vi "TL midbrain THINK.vi"(0 "Forebrain Comd":T2, 3 "error in":errorcluster, 4 "IR Sensors":T1) -> (5 "Behavior arrays":T3, 6 "Behavior\nVelocity OUT":dbl, 7 "error out":errorcluster)   [LabVIEW 2014]
doc: "This vi is the midbrain THINK routine. It selects the behaviors which the boat will use based upon the passed Forebrain Command."
uses:
  sensorsSTD.ctl
panel:
  out "Waveform Graph":cluster{dbl, dbl, dbl[][]}(graph)
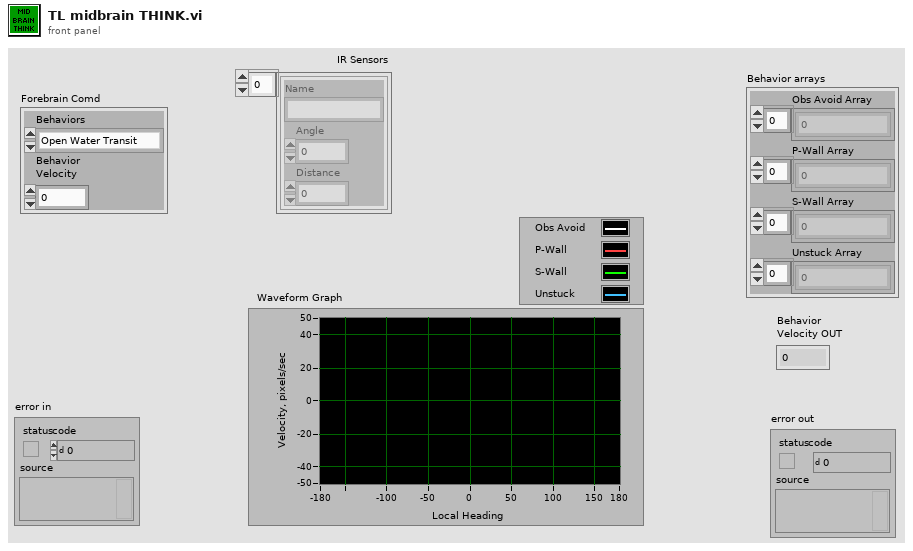
[diagram p1: front panel]
types:
  T1 = typedef "sensorsSTD.ctl" = cluster{"Name":string, "Angle":dbl, "Distance":dbl}[]
  T2 = cluster{"Behaviors":enum16{"Open Water Transit", "P-Wall Follow", "S-Wall Follow", "Get Unstuck"}, "Behavior\nVelocity":dbl}
  T3 = cluster{"Obs Avoid Array":dbl[], "P-Wall Array":dbl[], "S-Wall Array":dbl[], "Unstuck Array":dbl[]}
  T4 = enum16{"Open Water Transit", "P-Wall Follow", "S-Wall Follow", "Get Unstuck"}
  T5 = cluster{"Obstacle Avoidance":bool, "P-Wall Follow":bool, "S-Wall Follow":bool, "Get Unstuck":bool}
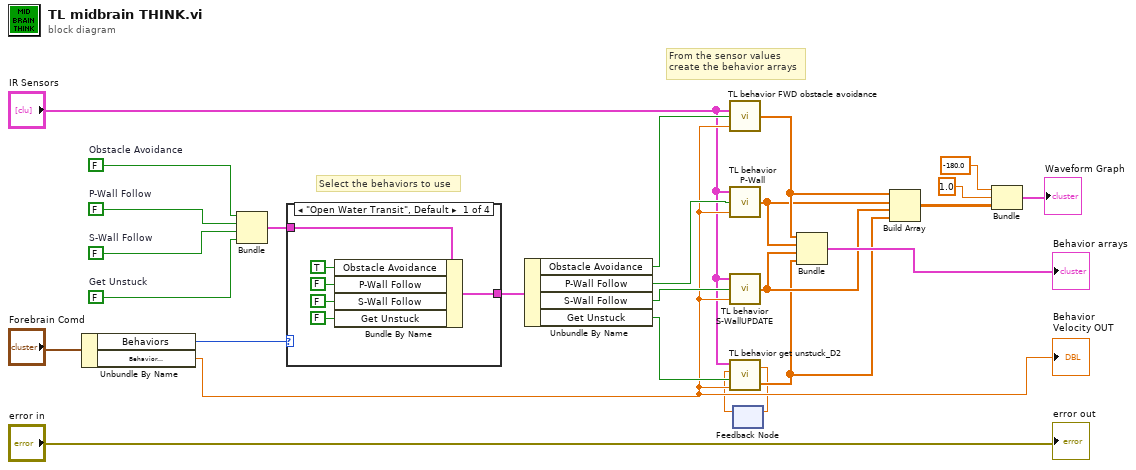
[diagram p0: block diagram]
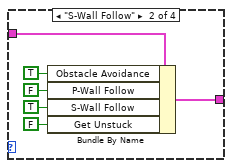
[diagram p2: hidden frame]
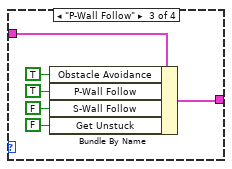
[diagram p3: hidden frame]
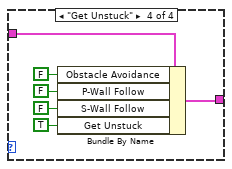
[diagram p4: hidden frame]
diagram:
  w22 = FALSE  # Get Unstuck
  w23 = FALSE  # S-Wall Follow
  w24 = FALSE  # P-Wall Follow
  w25 = FALSE  # Obstacle Avoidance
  # "From the sensor values\ncreate the behavior arrays"
  # "Select the behaviors to use"
  n1 = Unbundle By Name("Forebrain Comd") -> ("Behaviors"=w4:T4, "Behavior\nVelocity"=w14:dbl)
  "Behavior\nVelocity OUT" <- w14
  n2 = Bundle("Obstacle Avoidance"=w25, "P-Wall Follow"=w24, "S-Wall Follow"=w23, "Get Unstuck"=w22) -> (w21:T5)  [unwired: 1 in]
  n3 = case shown="\"Open Water Transit\", Default" w4 {
    tunnel: w21 -> [w32 w38 w44 w50]
    tunnel: [w30 w36 w42 w48] -> w20
    frame "Open Water Transit", Default {
      n4 = Bundle By Name(cluster=w32, "Obstacle Avoidance"=TRUE, "P-Wall Follow"=FALSE, "S-Wall Follow"=FALSE, "Get Unstuck"=FALSE) -> (w30:T5)
    }
    frame "S-Wall Follow" {
      n5 = Bundle By Name(cluster=w38, "Obstacle Avoidance"=TRUE, "P-Wall Follow"=FALSE, "S-Wall Follow"=TRUE, "Get Unstuck"=FALSE) -> (w36:T5)
    }
    frame "P-Wall Follow" {
      n6 = Bundle By Name(cluster=w44, "Obstacle Avoidance"=TRUE, "P-Wall Follow"=TRUE, "S-Wall Follow"=FALSE, "Get Unstuck"=FALSE) -> (w42:T5)
    }
    frame "Get Unstuck" {
      n7 = Bundle By Name(cluster=w50, "Obstacle Avoidance"=FALSE, "P-Wall Follow"=FALSE, "S-Wall Follow"=FALSE, "Get Unstuck"=TRUE) -> (w48:T5)
    }
  }
  n8 = Unbundle By Name(w20) -> ("Obstacle Avoidance"=w19:bool, "P-Wall Follow"=w16:bool, "S-Wall Follow"=w17:bool, "Get Unstuck"=w18:bool)
  n9 = call "TL behavior FWD obstacle avoidance.vi"("Behavior\nVelocity"=w14, "Activate?"=w19, "Sensor"="IR Sensors") -> ("Obs Avoid Array"=w10:dbl[])
  n10 = call "TL behavior P-Wall.vi"("Behavior\nVelocity"=w14, "Activate?"=w16, "Sensor"="IR Sensors") -> ("P-Wall Array"=w9:dbl[])
  n11 = call "TL behavior S-WallUPDATE.vi"("Behavior\nVelocity"=w14, "Activate?"=w17, "Sensor"="IR Sensors") -> ("S-Wall Array"=w7:dbl[])
  n12 = feedback #1() -> (w1:dbl)  [unwired: 1 in]
  n13 = call "TL behavior get unstuck_D2.vi"("Behavior\nVelocity"=w14, "Activate?"=w18, "Numeric"=w1, "Sensor"="IR Sensors") -> ("Unstuck Array"=w6:dbl[], "Numeric 2"=w2:dbl)
  n14 = feedback-in #1(w2) -> ()
  n15 = Bundle("Obs Avoid Array"=w10, "P-Wall Array"=w9, "S-Wall Array"=w7, "Unstuck Array"=w6) -> (→"Behavior arrays":T3)  [unwired: 1 in]
  n16 = Build Array(w10, w9, w7, w6) -> (w8:dbl[][])
  n17 = Bundle(-180.0, 1.0, w8) -> (→"Waveform Graph":cluster{dbl, dbl, dbl[][]})  [unwired: 1 in]
  "error out" <- "error in"
